vi "Extract M-S from Timestamp.vi"(10 "Waveform":waveform(dbl)) -> (1 "Time String":string, 2 "Elapsed Time (s)":dbl)   [LabVIEW 2012]
panel:
  out "date/time string":string
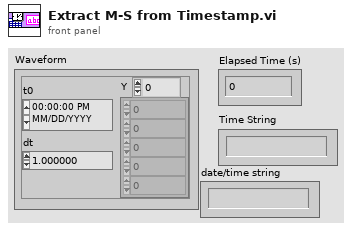
[diagram p1: front panel]
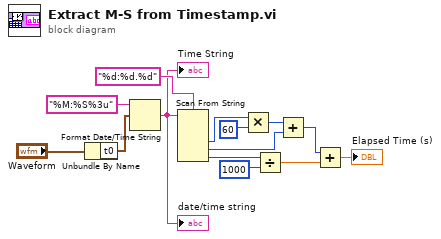
[diagram p0: block diagram]
diagram:
  n1 = Unbundle By Name("Waveform") -> ("t0"=w10:timestamp)
  n2 = Format Date/Time String(time format string (%c)="%M:%S%3u", seconds (now)=w10) -> (date/time string=w1:string)  [unwired: 1 in]
  "Time String" <- w1
  "date/time string" <- w1
  n3 = Scan From String(format string="%d:%d.%d", input string=w1) -> (output 1=w2:i32, output 2=w8:i32, output 3=w6:i32)  [unwired: 5 in, 3 out]
  n4 = Multiply(x=w2, y=60) -> (x*y=w12:i32)
  n5 = Divide(x=w6, y=1000) -> (x/y=w4:dbl)
  n6 = Add(x=w12, y=w8) -> (x+y=w7:i32)
  n7 = Add(x=w7, y=w4) -> (x+y=→"Elapsed Time (s)":dbl)
